vi "Decimate.vi"(6 "Select":enum16{"Pre DSP", "Post DSP"}(ring), 8 "error in (no error)":errorcluster, 11 "Instrument.DAQ":refnum<class "Instrument.DAQ.lvclass">) -> (0 "error out":errorcluster, 3 "Instrument.DAQ out":refnum<class "Instrument.DAQ.lvclass">)   [LabVIEW 2019, in "Instrument.Lockin.lvlib" / "Instrument.DAQ.lvclass"]
doc: "Decimates the input sequence X by the decimating factor and the averaging Boolean control."
uses:
  Instrument.DAQ.lvclass
  Instrument.DAQ.lvclass/Instrument.DAQ.ctl
  <vilib>/addons/Digital Filter Design/NI_DigFilterLicensed.lvlib
  <vilib>/addons/Digital Filter Design/_Objects.llb/DFD Multirate Filtering Mode.ctl
  <vilib>/measure/NI_MABase.lvlib
  <vilib>/addons/Digital Filter Design/_Objects.llb/DFD Multirate Filter Specification (Design).ctl
  <vilib>/addons/Digital Filter Design/Design.llb/DFD MRate Filter Design (Integer).vi
  <vilib>/addons/Digital Filter Design/Multirate.llb/DFD MRate Filtering (Wfm NChan).vi
  <vilib>/addons/Digital Filter Design/Multirate.llb/DFD NStage MRate Filtering (Wfm).vi
panel:
  out "x-y":dbl
  out "fs/2M":dbl
  in  "fpass":dbl
  in  "amplitude":dbl=1.0 format="%0.2p"
  in  "frequency":dbl=10.0 format="%0.2p"
  in  "sampling info":cluster{"Fs":dbl, "#s":dbl}={"Fs"=1000.0, "#s"=10000.0}
  in  "decimation":i32=4
  # "by Marco Tedaldi, Brain Research Institute, University of Zurich, 2013"
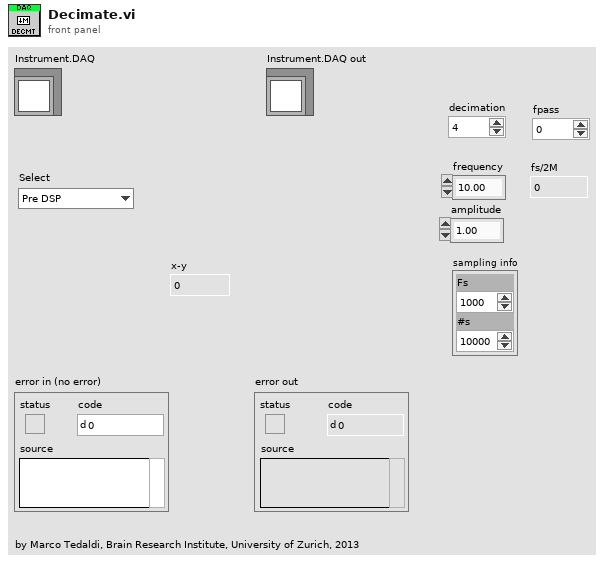
[diagram p1: front panel]
types:
  T1 = typedef "NI_DigFilterLicensed.lvlib/DFD Multirate Filter Specification (Design).ctl" = cluster{"fpass":dbl, "fstop":dbl}
  T2 = typedef "NI_DigFilterLicensed.lvlib/DFD Multirate Filtering Mode.ctl" = u16
  T3 = typedef "NI_DigFilterLicensed.lvlib/DFD Multirate Filter Obj.ctl" = cluster{"mMRate_Structure":enum16{"CIC", "FIR", "IIR", "Lattice"}, "mMRate_Mode":T4, "mMRate_Factor":i32, "mMRate_FIRParams":cluster{"mMRate_FIR_H":dbl[], "mMRate_FIR_IsNyquist?":bool, "mMRate_FIR_IsSymmetric?":bool}, "mMRate_CICParams":cluster{"mMRate_CIC_#Stage":i32, "mMRate_CIC_Lag":i32, "mMRate_CIC_Type":enum16{"Lowpass", "Highpass"}}, "mMRate_Order":i32, "mMRate_Version":string, "mMRate_Comments":string, "mMRate_RationalFactor":cluster{"mMRate_L":i32, "mMRate_M":i32}, "mMRate_Fs":dbl, "mMRate_Quantized?":bool, "mMRate_QFilterGain":dbl, "mMRate_CoefWl":i16, "mMRate_Scaling":cluster{"mMRate_ScaleByPowerOf2?":bool, "mMRate_ScaleType":T5}, "mMRate_InputWl":i16, "mMRate_OutputWl":i16, "mMRate_OutputMode":T6, "mMRate_MultMode":T7, "mMRate_BitPruning":bool, "mMRate_GainWl":i16, "mMRate_OutputFwl":i16, "mMRate_SumIwl":i16, "mMRate_InputIwl ":i16, "mMRate_SumWl":i16, "mMRate_CoefIwl":i16}
  T4 = typedef "NI_DigFilterLicensed.lvlib/DFD Multirate Mode.ctl" = i16
  T5 = typedef "NI_DigFilterLicensed.lvlib/DFD Coef Norm Type.ctl" = enum16{"No Norm", "Time Domain 1-Norm", "Time Domain 2-Norm", "Time Domain Inf-Norm"}
  T6 = typedef "NI_DigFilterLicensed.lvlib/DFD Round-off Mode.ctl" = enum16{"Nearest", "Truncation"}
  T7 = typedef "NI_DigFilterLicensed.lvlib/DFD FXP MRate Multiply Mode.ctl" = enum16{"Truncated", "Full"}
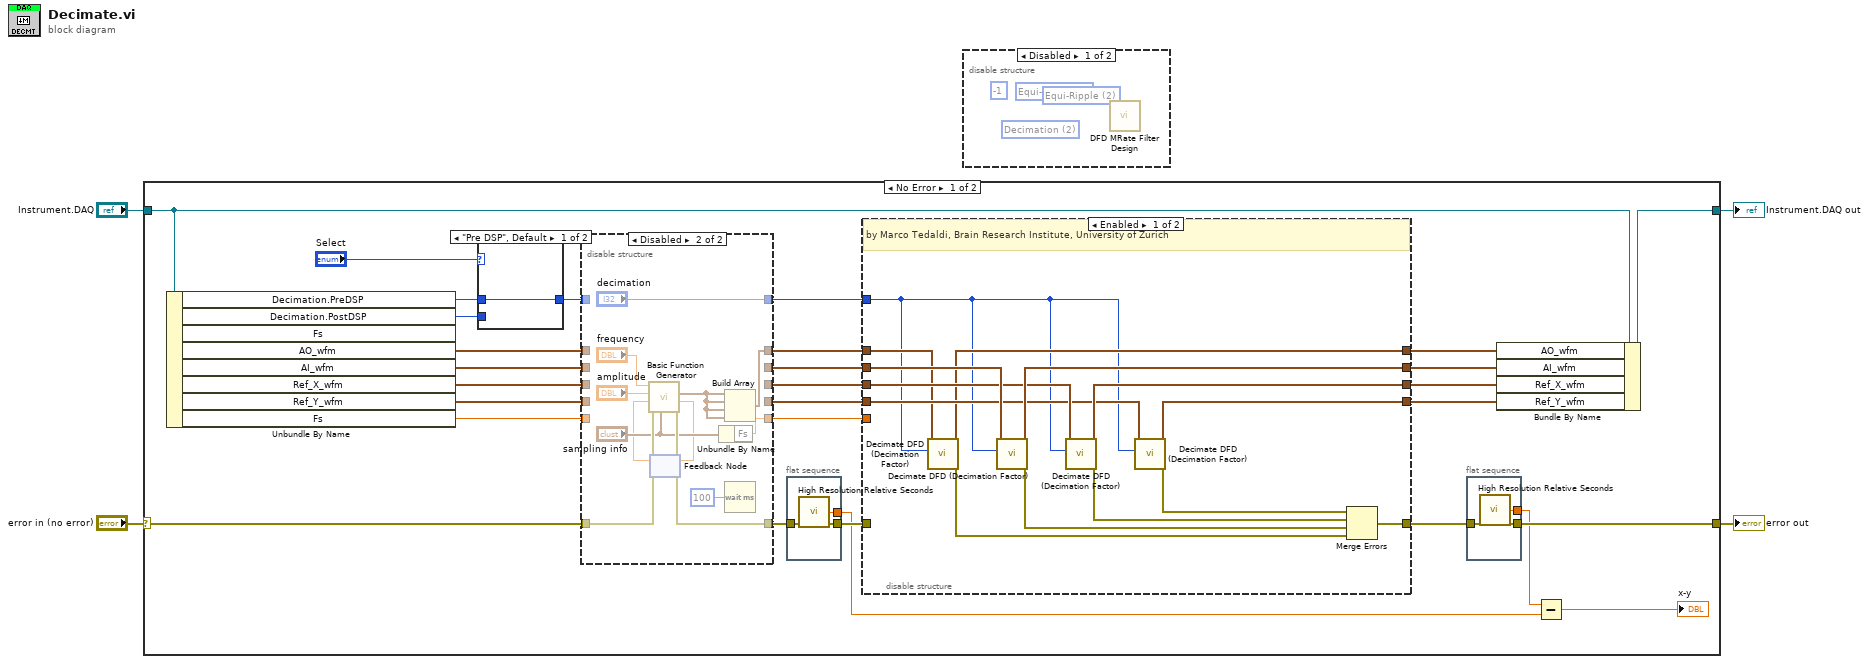
[diagram p0: block diagram]
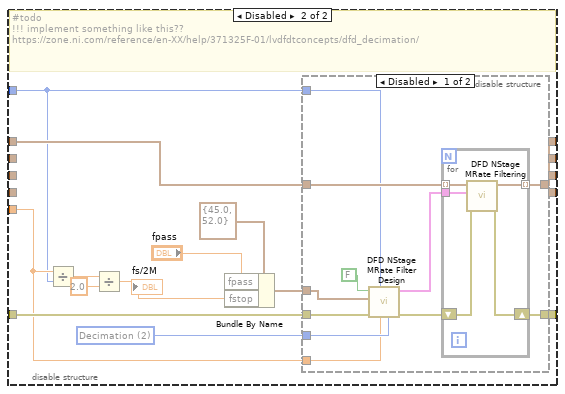
[diagram p4: hidden frame]
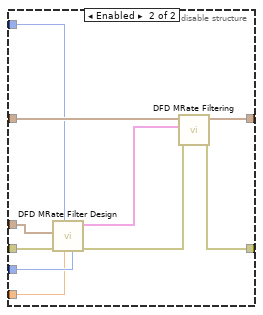
[diagram p5: hidden frame]
diagram:
  n1 = case shown="No Error" "error in (no error)" {
    selector: "error in (no error)" -> [w26 w113]
    tunnel: [w29 w113] -> w4
    tunnel: "Instrument.DAQ" -> [w25 w112]
    tunnel: [w24 w112] -> w1
    frame No Error {
      n2 = Unbundle By Name(w25) -> ("Decimation.PreDSP"=w19:i32, "Decimation.PostDSP"=w18:i32, "AO_wfm"=w16:waveform(dbl)[], "AI_wfm"=w11:waveform(dbl)[], "Ref_X_wfm"=w9:waveform(dbl)[], "Ref_Y_wfm"=w6:waveform(dbl)[], "Fs"=w5:dbl)  [unwired: 1 out]
      n3 = case shown="\"Pre DSP\", Default" "Select" {
        tunnel: [w34 w35] -> w20
        tunnel: w19 -> [w34 _]
        tunnel: w18 -> [_ w35]
        frame "Pre DSP", Default {
        }
        frame "Post DSP" {
        }
      }
      n4 = disable-structure shown="Disabled" {
        disable-tunnel: [w46 w58] -> w32
        disable-tunnel: w5 -> [w46 _]
        disable-tunnel: [w43 "decimation"] -> w31
        disable-tunnel: w16 -> [w45 _]
        disable-tunnel: [w45 w49] -> w17
        disable-tunnel: w26 -> [w44 w54]
        disable-tunnel: [w44 w53] -> w23
        disable-tunnel: w20 -> [w43 _]
        disable-tunnel: w11 -> [w42 _]
        disable-tunnel: [w42 _] -> w10
        disable-tunnel: w9 -> [w41 _]
        disable-tunnel: [w41 _] -> w8
        disable-tunnel: [w40 _] -> w7
        disable-tunnel: w6 -> [w40 _]
        frame Enabled {
        }
        frame Disabled {
          n5 = feedback #1() -> (w51:dbl)  [unwired: 1 in]
          n6 = call <vilib>:"Basic Function Generator.vi"("sampling info"="sampling info", "error in (no error)"=w54, "phase"=w51, "amplitude"="amplitude", "frequency"="frequency") -> ("error out"=w53:errorcluster, "phase out"=w50:dbl, "signal out"=w47:waveform(dbl))  [unwired: 4 in]
          n7 = feedback-in #1(w50) -> ()
          n8 = Unbundle By Name("sampling info") -> ("Fs"=w58:dbl)
          n9 = Build Array(w47, w47, w47, w47) -> (w49:waveform(dbl)[])
          n10 = Wait (ms)(milliseconds to wait=u32 100) -> ()  [unwired: 1 out]
        }
      }
      n11 = flat-sequence {
        tunnel: [w39] -> w30
        tunnel: w23 -> [w39]
        tunnel: [w38] -> w28
        frame #0 {
          n12 = call <vilib>:"High Resolution Relative Seconds.vi"() -> ("relative seconds"=w38:dbl)
        }
      }
      n13 = disable-structure shown="Enabled" {
        disable-tunnel: w30 -> [_ w82]
        disable-tunnel: [w60 w83] -> w15
        disable-tunnel: [w66 w85] -> w33
        disable-tunnel: w17 -> [w61 w84]
        disable-tunnel: w31 -> [w59 w77]
        disable-tunnel: w32 -> [_ w80]
        disable-tunnel: w10 -> [w72 _]
        disable-tunnel: [w71 _] -> w14
        disable-tunnel: w8 -> [w70 _]
        disable-tunnel: [w69 _] -> w13
        disable-tunnel: w7 -> [w68 _]
        disable-tunnel: [w67 _] -> w12
        frame Enabled {
          # "by Marco Tedaldi, Brain Research Institute, University of Zurich"
          n14 = call "Decimate DFD (Decimation Factor).vi"("Decimation Factor"=w59, "Waveforms in"=w61) -> ("error out"=w62:errorcluster, "waveforms out"=w60:waveform(dbl)[])  [unwired: 8 in]
          n15 = call "Decimate DFD (Decimation Factor).vi"("Decimation Factor"=w59, "Waveforms in"=w72) -> ("error out"=w63:errorcluster, "waveforms out"=w71:waveform(dbl)[])  [unwired: 8 in]
          n16 = call "Decimate DFD (Decimation Factor).vi"("Decimation Factor"=w59, "Waveforms in"=w70) -> ("error out"=w64:errorcluster, "waveforms out"=w69:waveform(dbl)[])  [unwired: 8 in]
          n17 = call "Decimate DFD (Decimation Factor).vi"("Decimation Factor"=w59, "Waveforms in"=w68) -> ("error out"=w65:errorcluster, "waveforms out"=w67:waveform(dbl)[])  [unwired: 8 in]
          n18 = Merge Errors(w65, w64, w63, w62) -> (w66:errorcluster)
        }
        frame Disabled {
          w81 = T2 2 items=["No Rate Change", "Interpolation", "Decimation"] ("filtering mode")
          # "#todo\n!!! implement something like this??\nhttps://zone.ni.com/reference/en-XX/help/371325F-01/lvdfdtconcepts/dfd_decimation/"
          n19 = Divide(x=w80, y=w77) -> (x/y=w76:dbl)
          n20 = Divide(x=w76, y=2.0) -> (x/y=w74:dbl)
          "fs/2M" <- w74
          n21 = Bundle By Name(cluster=T1 {"fpass"=45.0, "fstop"=52.0} ("freq specs [Hz]"), "fpass"="fpass", "fstop"=w74) -> (w73:T1)
          n22 = disable-structure shown="Disabled" {
            disable-tunnel: [w96 w103] -> w85
            disable-tunnel: w84 -> [w95 w107]
            disable-tunnel: [w94 w105] -> w83
            disable-tunnel: w82 -> [w93 w111]
            disable-tunnel: w81 -> [w91 w109]
            disable-tunnel: w80 -> [w88 w108]
            disable-tunnel: w77 -> [w87 w102]
            disable-tunnel: w73 -> [w86 w110]
            frame Disabled {
              n23 = call <vilib>:"DFD NStage MRate Filter Design.vi"("filtering mode"=w91, "fs in [Hz]"=w88, "factor"=w87, "error in (no error)"=w93, "freq specs [Hz]"=w86, "using CIC?"=FALSE) -> ("error out"=w92:errorcluster, "multirate filters out"=w90:T3[])  [unwired: 4 in]
              n24 = for {
                tunnel: w95 -> [w99] mode=indexing
                tunnel: [w98] -> w94 mode=indexing
                tunnel: w90 -> [w97]
                shift-right: [w101] -> w96
                shift-left: w92 -> [w100]
                n25 = call-poly <vilib>:"DFD NStage MRate Filtering.vi"("error in (no error)"=w100, "multirate filters"=w97, "signal in"=w99) -> ("error out"=w101:errorcluster, "signal out"=w98:waveform(dbl))  [unwired: 7 in]
              }
            }
            frame Enabled {
              n26 = call-poly <vilib>:"DFD MRate Filter Design.vi"("filtering mode"=w109, "fs in [Hz]"=w108, "factor"=w102, "error in (no error)"=w111, "freq specs [Hz]"=w110) -> ("error out"=w104:errorcluster, "multirate filter out"=w106:T3)  [unwired: 5 in]
              n27 = call-poly <vilib>:"DFD MRate Filtering.vi"("error in (no error)"=w104, "multirate filter"=w106, "signal in"=w107) -> ("error out"=w103:errorcluster, "signal out"=w105:waveform(dbl)[])  [unwired: 7 in]
            }
          }
        }
      }
      n28 = flat-sequence {
        tunnel: [w37] -> w29
        tunnel: w33 -> [w37]
        tunnel: [w36] -> w22
        frame #0 {
          n29 = call <vilib>:"High Resolution Relative Seconds.vi"() -> ("relative seconds"=w36:dbl)
        }
      }
      n30 = Bundle By Name(cluster=w25, "AO_wfm"=w15, "AI_wfm"=w14, "Ref_X_wfm"=w13, "Ref_Y_wfm"=w12) -> (w24:refnum<class "Instrument.DAQ.lvclass">)
      n31 = Subtract(x=w22, y=w28) -> (x-y=→"x-y":dbl)
    }
    frame Error {
    }
  }
  "error out" <- w4
  "Instrument.DAQ out" <- w1
  n32 = disable-structure shown="Disabled" {
    frame Disabled {
      (unwired) -1 ("order")
      (unwired) u16 2 items=["Kaiser Window", "Dolph-Chebyshev Window", "Equi-Ripple"] ("method")
      w114 = u16 2 items=["Kaiser Window", "Dolph-Chebyshev Window", "Equi-Ripple"] ("method")
      (unwired) T2 2 items=["No Rate Change", "Interpolation", "Decimation"] ("filtering mode")
      n33 = call-poly <vilib>:"DFD MRate Filter Design.vi"() -> ()  [unwired: 10 in, 2 out]
    }
    frame Enabled {
    }
  }
